vi "Main.vi"() -> ()   [LabVIEW 2020]
doc: "Use this template to build a simple state machine design pattern. Each state executes code and determines which state to transition to."
uses:
  controls/State.ctl
  controls/Data.ctl
  VirtualLab.lvlibp/VISASimulator/VISALib.lvlib
panel:
  in  "Do Something Else <Replace Me>":bool
  in  "Do Something <Replace Me>":bool
  in  "Exit":bool
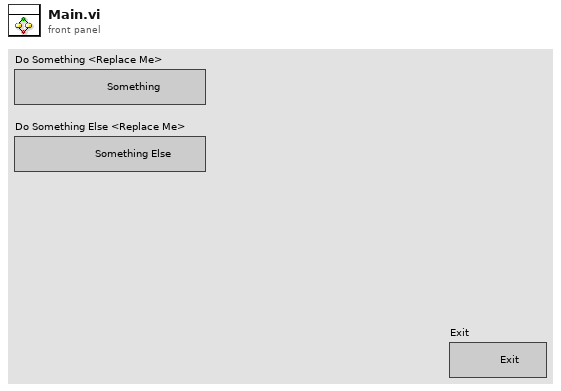
[diagram p1: front panel]
types:
  T1 = typedef "Data.ctl" = cluster{"Boolean <Replace Me>":bool, "String <Replace Me>":string, "Numeric <Replace Me>":dbl}
  T2 = typedef "State.ctl" = enum16{"Initialize", "Wait for Event", "User State 1", "User State 2", "Exit"}
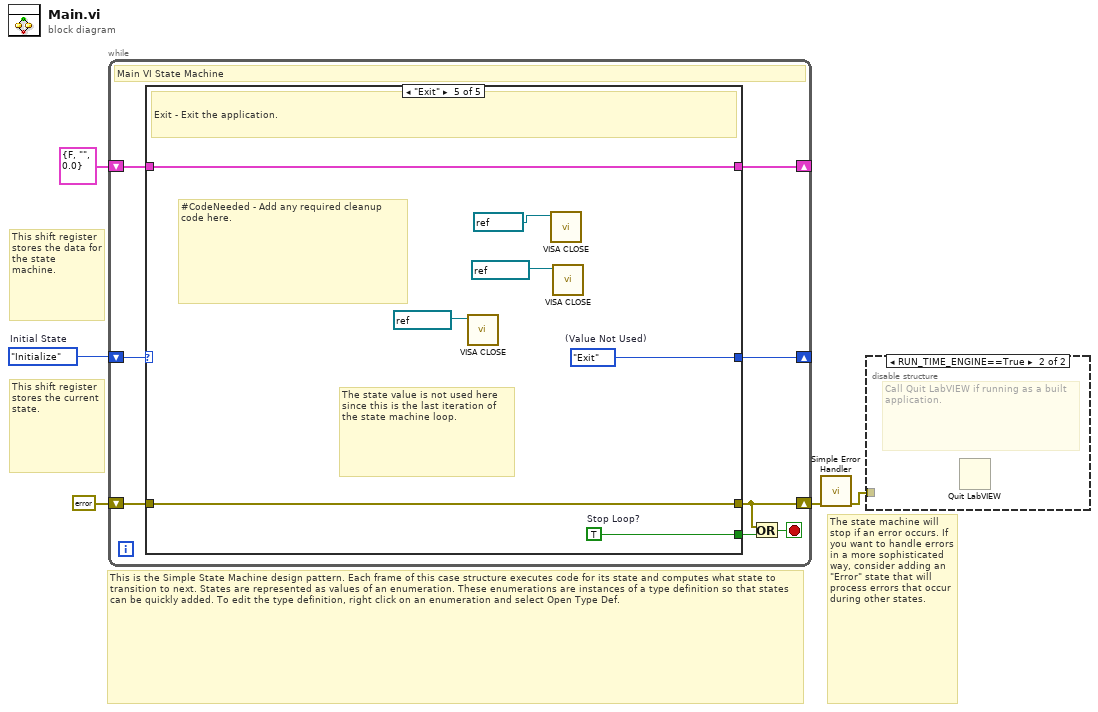
[diagram p0: block diagram]
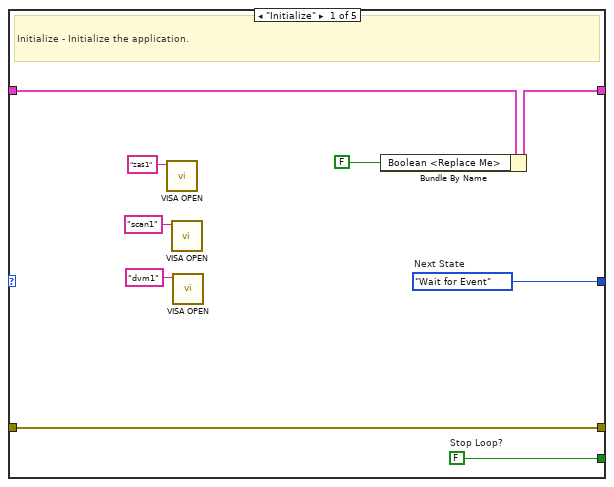
[diagram p3: hidden frame]
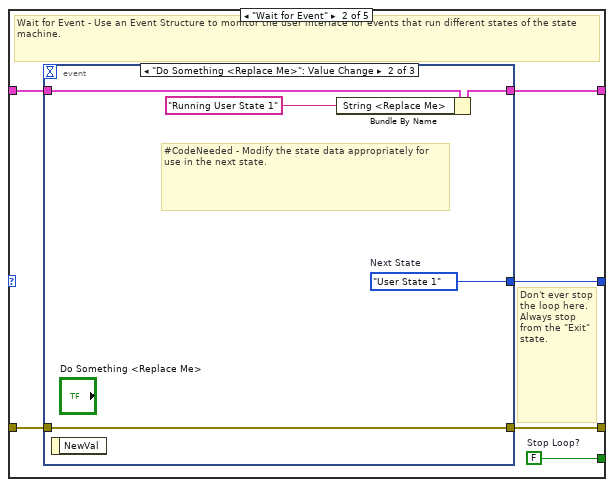
[diagram p4: hidden frame]
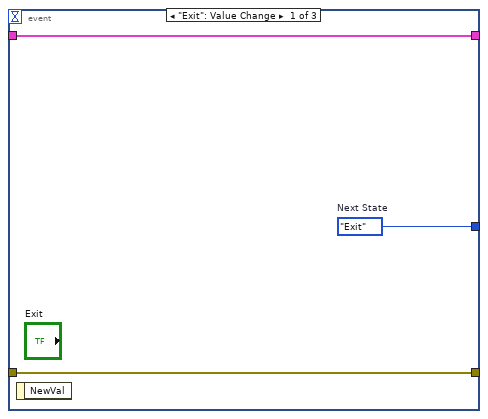
[diagram p5: hidden frame]
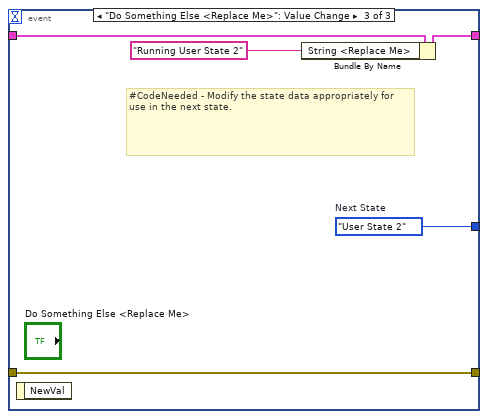
[diagram p6: hidden frame]
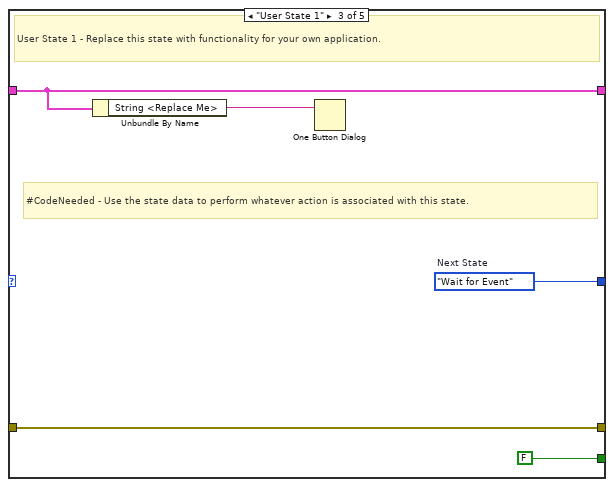
[diagram p7: hidden frame]
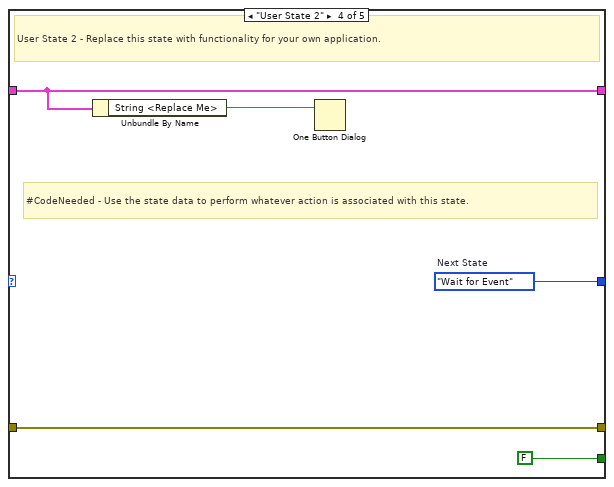
[diagram p8: hidden frame]
diagram:
  w5 = State."Initialize"  # Initial State
  # "The state machine will stop if an error occurs. If you want to handle errors in a more sophisticated way, consider adding an \"Error\" state that will process errors that occur during other states."
  # "This shift register stores the data for the state machine."
  # "This is the Simple State Machine design pattern. Each frame of this case structure executes code for its state and computes what state to transition to next. States are represented as values of an enumeration. These enumerations are instances of a type definition so that states can be quickly added. To edit the type definition, right click on an enumeration and select Open Type Def."
  # "This shift register stores the current state."
  n1 = while {
    shift-right: [w12] -> _
    shift-left: w5 -> [w13]
    shift-right: [w10] -> _
    shift-left: T1 {"Boolean <Replace Me>"=FALSE, "String <Replace Me>"="", "Numeric <Replace Me>"=0.0} ("Data") -> [w11]
    shift-right: [w6] -> w2
    shift-left: errorcluster {"status"=FALSE, "code"=0, "source"=""} ("error constant") -> [w9]
    stop <- w7 stop-if-true
    # "Main VI State Machine"
    n2 = case shown="\"Exit\"" w13 {
      tunnel: [w22 w28 w46 w51 w58] -> w12
      tunnel: [w21 w27 FALSE ("Stop Loop?") FALSE ("Stop Loop?") w56] -> w8
      tunnel: w11 -> [w20 w26 w44 w49 w57]
      tunnel: [w19 w25 w44 w49 w57] -> w10
      tunnel: w9 -> [w17 w24 w42 w47 w55]
      tunnel: [w17 w23 w42 w47 w55] -> w6
      frame "Initialize" {
        w21 = FALSE  # Stop Loop?
        w22 = State."Wait for Event"  # Next State
        # "Initialize - Initialize the application."
        n3 = call "VISA OPEN.vi"("VISA resource name"="zas1") -> ()  [unwired: 9 in, 2 out]
        n4 = call "VISA OPEN.vi"("VISA resource name"="scan1") -> ()  [unwired: 9 in, 2 out]
        n5 = call "VISA OPEN.vi"("VISA resource name"="dvm1") -> ()  [unwired: 9 in, 2 out]
        n6 = Bundle By Name(cluster=w20, "Boolean <Replace Me>"=FALSE ("Replace_Me_Boolean")) -> (w19:T1)
      }
      frame "Wait for Event" {
        w27 = FALSE  # Stop Loop?
        # "Don't ever stop the loop here. Always stop from the \"Exit\" state."
        # "Wait for Event - Use an Event Structure to monitor the user interface for events that run different states of the state machine."
        n7 = event shown="[1] \"Do Something <Replace Me>\": Value Change" {
          selector: _ -> [_ _ _]
          dyn-events: _ -> [_ _ _]
          timeout: _ -> [_ _ _]
          tunnel: [w31 w36 w41] -> w28
          tunnel: w26 -> [w30 w35 w40]
          tunnel: [w30 w34 w39] -> w25
          tunnel: w24 -> [w29 w32 w37]
          tunnel: [w29 w32 w37] -> w23
          event "Exit": Value Change {
            w31 = State."Exit"  # Next State
            n8 = event-data() -> ()  [unwired: 1 in, 1 out]
          }
          event "Do Something <Replace Me>": Value Change {
            w36 = State."User State 1"  # Next State
            # "#CodeNeeded - Modify the state data appropriately for use in the next state."
            n9 = event-data() -> ()  [unwired: 1 in, 1 out]
            n10 = Bundle By Name(cluster=w35, "String <Replace Me>"="Running User State 1" ("Running User State 1")) -> (w34:T1)
          }
          event "Do Something Else <Replace Me>": Value Change {
            w41 = State."User State 2"  # Next State
            # "#CodeNeeded - Modify the state data appropriately for use in the next state."
            n11 = event-data() -> ()  [unwired: 1 in, 1 out]
            n12 = Bundle By Name(cluster=w40, "String <Replace Me>"="Running User State 2" ("Running User State 2")) -> (w39:T1)
          }
        }
      }
      frame "User State 1" {
        w46 = State."Wait for Event"  # Next State
        # "#CodeNeeded - Use the state data to perform whatever action is associated with this state."
        # "User State 1 - Replace this state with functionality for your own application."
        n13 = Unbundle By Name(w44) -> ("String <Replace Me>"=w43:string)
        n14 = One Button Dialog(message=w43) -> ()  [unwired: 1 in, 1 out]
      }
      frame "User State 2" {
        w51 = State."Wait for Event"  # Next State
        # "#CodeNeeded - Use the state data to perform whatever action is associated with this state."
        # "User State 2 - Replace this state with functionality for your own application."
        n15 = Unbundle By Name(w49) -> ("String <Replace Me>"=w48:string)
        n16 = One Button Dialog(message=w48) -> ()  [unwired: 1 in, 1 out]
      }
      frame "Exit" {
        w56 = TRUE  # Stop Loop?
        w58 = State."Exit"  # (Value Not Used)
        # "#CodeNeeded - Add any required cleanup code here."
        # "The state value is not used here since this is the last iteration of the state machine loop."
        # "Exit - Exit the application."
        n17 = call "VISA CLOSE.vi"("VISA resource name"=refnum<visa-resource-name> "dvm1") -> ()  [unwired: 10 in, 1 out]
        n18 = call "VISA CLOSE.vi"("VISA resource name"=refnum<visa-resource-name> "zas1") -> ()  [unwired: 10 in, 1 out]
        n19 = call "VISA CLOSE.vi"("VISA resource name"=refnum<visa-resource-name> "scan1") -> ()  [unwired: 10 in, 1 out]
      }
    }
    n20 = Or(x=w6, y=w8) -> (x .or. y?=w7:bool)
  }
  n21 = call <vilib>:"Simple Error Handler.vi"("error in (no error)"=w2) -> ("error out"=w1:errorcluster)  [unwired: 4 in, 4 out]
  n22 = disable-structure shown="RUN_TIME_ENGINE==True" {
    disable-tunnel: w1 -> [_ _]
    frame condition #0 (active) {
    }
    frame condition #1 {
      # "Call Quit LabVIEW if running as a built application."
      n23 = Quit LabVIEW() -> ()  [unwired: 1 in]
    }
  }
